vi "Helper - Export - Square.vi"() -> (3 "Square with Noise":dbl[](array[numeric]))   [LabVIEW 2023]
doc: "Generates a Square signal with noise."
panel:
  # "Generates a Square signal with noise."
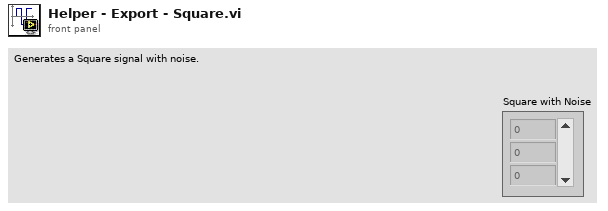
[diagram p1: front panel]
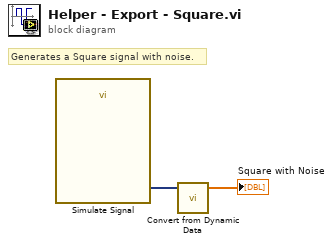
[diagram p0: block diagram]
diagram:
  # "Generates a Square signal with noise."
  n1 = call "Simulate Signal"() -> ("Square with Uniform Noise"=w2:dynamicdata)  [unwired: 14 in, 1 out]
  n2 = call "Convert from Dynamic Data"("Dynamic Data Type"=w2) -> ("Array"=→"Square with Noise":dbl[])  [unwired: 3 in]
